vi "Get Waveform and Sample.vi"(11 "Acquired Data":T1) -> (2 "As scalar":dbl, 3 "Waveform":waveform(dbl))   [LabVIEW 2021, in "Settings.lvlib"]
uses:
  Settings.lvlib
  Acquisition/Acquired Data.ctl
  Acquisition/Acquisition.lvlib
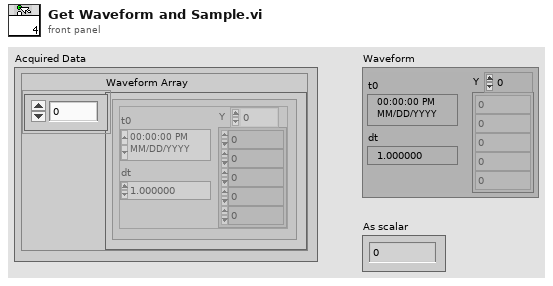
[diagram p1: front panel]
types:
  T1 = typedef "Acquisition.lvlib/Acquired Data.ctl" = cluster{"Waveform Array":waveform(dbl)[]}
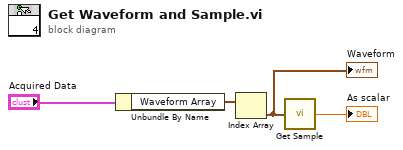
[diagram p0: block diagram]
diagram:
  n1 = Unbundle By Name("Acquired Data") -> ("Waveform Array"=w3:waveform(dbl)[])
  n2 = Index Array(array=w3) -> (element=w4:waveform(dbl))  [unwired: 1 in]
  "Waveform" <- w4
  n3 = call "Get Sample.vi"("Waveform"=w4) -> ("As scalar"=→"As scalar":dbl)
